vi "STOP_FGV.vi"(10 "Input":bool, 11 "Enum":enum16{"Read", "Write"}(ring)) -> (2 "Output":bool)   [LabVIEW 2018]
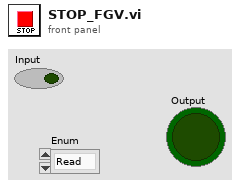
[diagram p1: front panel]
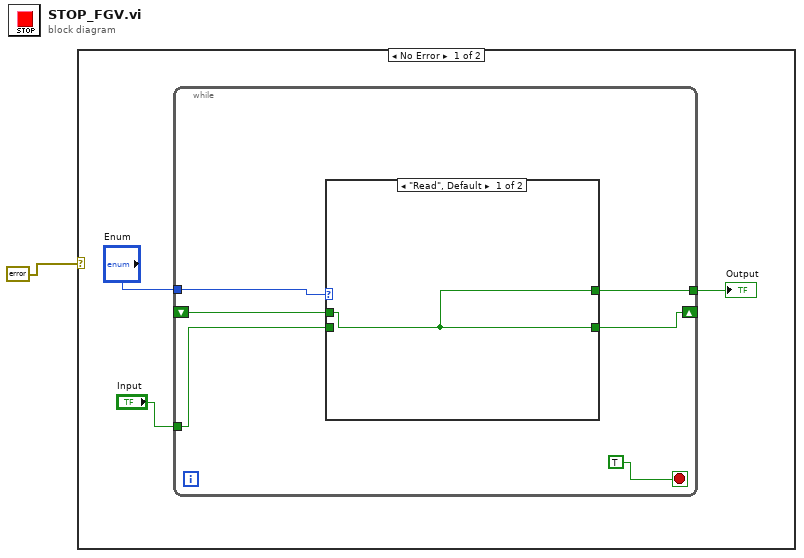
[diagram p0: block diagram]
diagram:
  n1 = case shown="No Error" errorcluster {"status"=FALSE, "code"=0, "source"=""} ("error constant") {
    frame No Error {
      n2 = while {
        tunnel: "Enum" -> [w10]
        tunnel: "Input" -> [w8]
        shift-right: [w9] -> _
        shift-left: _ -> [w6]
        tunnel: [w7] -> w2
        stop <- TRUE stop-if-true
        n3 = case shown="\"Read\", Default" w10 {
          tunnel: [w11 w12] -> w9
          tunnel: w8 -> [_ w12]
          tunnel: [w11 w12] -> w7
          tunnel: w6 -> [w11 _]
          frame "Read", Default {
          }
          frame "Write" {
          }
        }
      }
      "Output" <- w2
    }
    frame Error {
    }
  }
